vi "VCS Export Parameter.vi"(6 "error in (no error)":errorcluster, 8 "export":T1 {"showMsg" items=["false", "true"]; "showDlg" items=["false", "true"]}, 9 "axis in":cluster{"keyHandle":u32, "nodeId":u16}={"keyHandle"=0, "nodeId"=1}) -> (0 "error out":errorcluster, 3 "axis out":cluster{"keyHandle":u32, "nodeId":u16}={"keyHandle"=0, "nodeId"=1})   [LabVIEW 2017, in "maxonEPOS.lvlib"]
doc: "<B>VCS_ExportParameter</B> reads all parameters of the device and writes this into the file."
uses:
  Examples/maxonEPOS.lvlib
  SSI_Tool/InstrumentsInterfaces/Motordriver/maxon EPOS/Resources/EposCmd.dll
  SSI_Tool/InstrumentsInterfaces/Motordriver/maxon EPOS/Resources/EposCmd64.dll
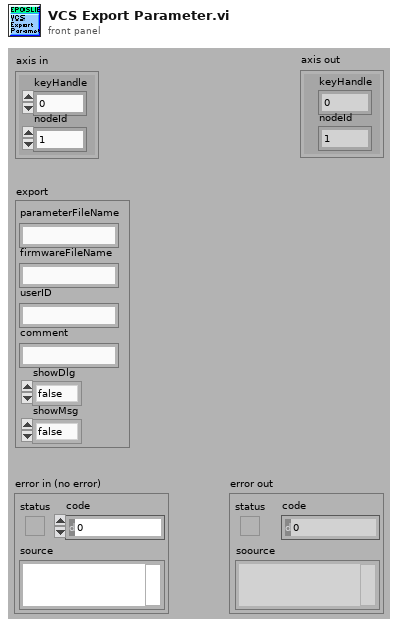
[diagram p1: front panel]
types:
  T1 = cluster{"parameterFileName":string, "firmwareFileName":string, "userID":string, "comment":string, "showDlg":i32, "showMsg":i32}
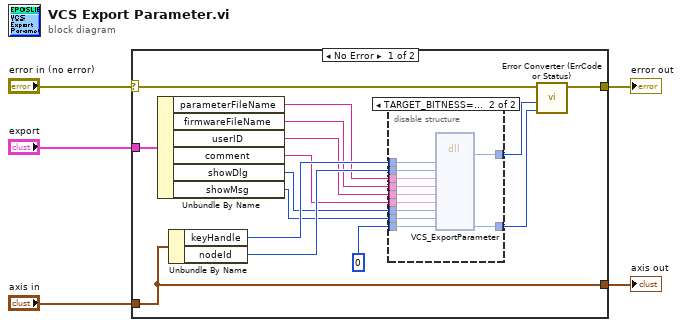
[diagram p0: block diagram]
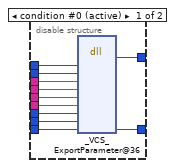
[diagram p2: hidden frame]
diagram:
  n1 = case shown="No Error" "error in (no error)" {
    selector: "error in (no error)" -> [w18 w43]
    tunnel: "axis in" -> [w20 w44]
    tunnel: [w20 w44] -> w4
    tunnel: [w19 w43] -> w3
    tunnel: "export" -> [w12 _]
    frame No Error {
      n2 = Unbundle By Name(w12) -> ("parameterFileName"=w11:string, "firmwareFileName"=w10:string, "userID"=w9:string, "comment"=w8:string, "showDlg"=w7:i32, "showMsg"=w6:i32)
      n3 = Unbundle By Name(w20) -> ("keyHandle"=w14:u32, "nodeId"=w13:u16)
      n4 = disable-structure shown="TARGET_BITNESS==64" {
        disable-tunnel: u32 0 ("pErrorCode") -> [w31 w42]
        disable-tunnel: [w30 w41] -> w16
        disable-tunnel: [w29 w40] -> w15
        disable-tunnel: w14 -> [w28 w39]
        disable-tunnel: w13 -> [w27 w38]
        disable-tunnel: w11 -> [w26 w37]
        disable-tunnel: w10 -> [w25 w36]
        disable-tunnel: w9 -> [w24 w35]
        disable-tunnel: w8 -> [w23 w34]
        disable-tunnel: w7 -> [w22 w33]
        disable-tunnel: w6 -> [w21 w32]
        frame condition #0 (active) {
          n5 = dll-call lib="C:/workspace/project/scancon/sw/SSI_Tool/InstrumentsInterfaces/Motordriver/maxon EPOS/Resources/EposCmd.*" fn="_VCS_ExportParameter@36"("KeyHandle"=w28, "NodeId"=w27, "pParameterFileName"=w26, "pBinaryFile"=w25, "pUserID"=w24, "pComment"=w23, "ShowDlg"=w22, "ShowMsg"=w21, "pErrorCode"=w31) -> (w29:i32, "pErrorCode"=w30:u32)  [unwired: 11 in, 2 out]
        }
        frame condition #1 {
          n6 = dll-call lib="C:/setup/Resources/EposCmd64.*" fn="VCS_ExportParameter" ("EposCmd.dll:_VCS_ExportParameter@36")("KeyHandle"=w39, "NodeId"=w38, "pParameterFileName"=w37, "pBinaryFile"=w36, "pUserID"=w35, "pComment"=w34, "ShowDlg"=w33, "ShowMsg"=w32, "pErrorCode"=w42) -> ("Rückgabetyp"=w40:i32, "pErrorCode"=w41:u32)  [unwired: 11 in, 2 out]
        }
      }
      n7 = call "Error Converter (ErrCode or Status).vi"("error code"=w16, "return type"=w15, "error in (no error)"=w18) -> ("error out"=w19:errorcluster)  [unwired: 7 in]
    }
    frame Error {
    }
  }
  "error out" <- w3
  "axis out" <- w4
